vi "Send ADC.vi"(8 "error in (no error)":errorcluster, 9 "Channel":enum16{""}(ring), 10 "VISA resource name":refnum<visa-resource-name>, 11 "NXP in":refnum<class "NXP.lvclass">) -> (0 "error out":errorcluster, 1 "Response":i32, 2 "VISA resource name 2":refnum<visa-resource-name>, 3 "NXP out":refnum<class "NXP.lvclass">)   [LabVIEW 2020, in "NXP.lvclass"]
uses:
  NXP.lvclass
  40103fee-a46f-41e1-b92f-718061ddcfe4.vi
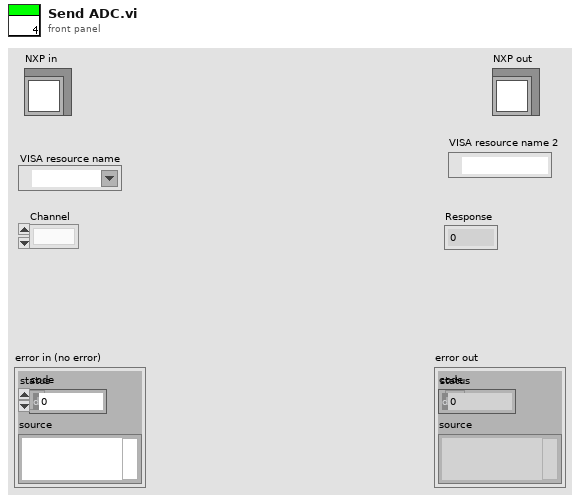
[diagram p1: front panel]
types:
  T1 = enum16{"Write", "Read", "Config", "Reset", "Close"}
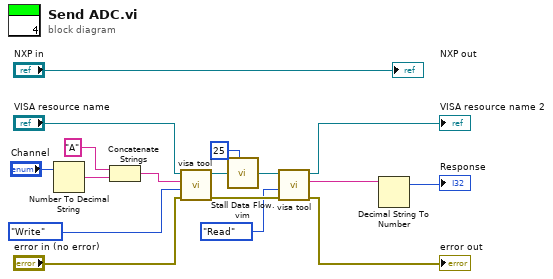
[diagram p0: block diagram]
diagram:
  n1 = Number To Decimal String(number="Channel") -> (decimal integer string=w11:string)  [unwired: 1 in]
  n2 = Concatenate Strings("A" ("string"), w11) -> (w10:string)
  n3 = call "visa tool.vi"("error in (no error)"="error in (no error)", "Opciones"=T1."Write", "Write"=w10, "VISA com port"="VISA resource name") -> ("error out"=w4:errorcluster, "VISA com port 2"=w8:refnum<visa-resource-name>)  [unwired: 5 in, 1 out]
  n4 = call "Stall Data Flow.vim"("value in"=w8, "milliseconds to wait"=u32 25) -> ("value out"=w7:refnum<visa-resource-name>)  [unwired: 1 out]
  n5 = call "visa tool.vi"("error in (no error)"=w4, "Opciones"=T1."Read", "VISA com port"=w7) -> ("error out"=→"error out":errorcluster, "Read"=w3:string, "VISA com port 2"=→"VISA resource name 2":refnum<visa-resource-name>)  [unwired: 6 in]
  n6 = Decimal String To Number(string=w3) -> (offset past number=→"Response":i32)  [unwired: 2 in, 1 out]
  "NXP out" <- "NXP in"
